vi "Open Workbook.vi"(7 "Create if does not exist? (T)":bool=TRUE, 8 "error in (no error)":errorcluster, 10 "File Name":path) -> (0 "error out":errorcluster, 3 "Workbook Reference Out":refnum<k24>)   [LabVIEW 2013]
uses:
  C:/PhaeronGit/LVNPOI/Resources/NPOI 2.1.1 dotnet2/NPOI.dll
  Resources/NPOI 2.1.1 dotnet2/NPOI.dll
  <vilib>/Utility/error.llb/Error Cluster From Error Code.vi
  <vilib>/ErrorRing/Error Ring.xnode
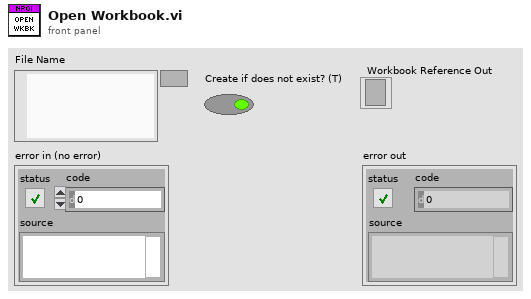
[diagram p1: front panel]
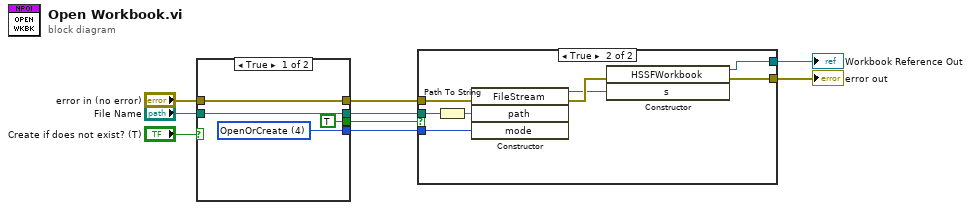
[diagram p0: block diagram]
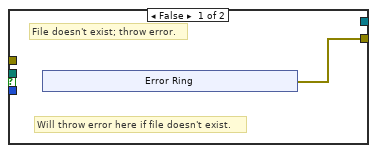
[diagram p2: hidden frame]
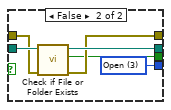
[diagram p3: hidden frame]
diagram:
  n1 = case shown="True" "Create if does not exist? (T)" {
    tunnel: [w13 w19] -> w7
    tunnel: [w12 w15] -> w6
    tunnel: "error in (no error)" -> [w12 w16]
    tunnel: [w11 w17] -> w4
    tunnel: "File Name" -> [w11 w18]
    tunnel: [TRUE ("file or folder exists?") w14] -> w1
    frame True {
      w13 = 4 items=["CreateNew"=1, "Create"=2, "Open"=3, "OpenOrCreate"=4, "Truncate"=5, "Append"=6] ("mode")
    }
    frame False {
      w19 = 3 items=["CreateNew"=1, "Create"=2, "Open"=3, "OpenOrCreate"=4, "Truncate"=5, "Append"=6] ("mode")
      n2 = call <vilib>:"Check if File or Folder Exists.vi"("error in (no error)"=w16, "path"=w18) -> ("error out"=w15:errorcluster, "file or folder exists?"=w14:bool, "dup path"=w17:path)  [unwired: 7 in]
    }
  }
  n3 = case shown="True" w1 {
    tunnel: [_ w30] -> w9
    tunnel: [w20 w29] -> w8
    tunnel: w7 -> [_ w28]
    tunnel: w6 -> [_ w27]
    tunnel: w4 -> [_ w26]
    frame False {
      # "File doesn't exist; throw error."
      # "Will throw error here if file doesn't exist."
      n4 = xnode "Error Ring"() -> ("error out"=w20:errorcluster)
    }
    frame True {
      n5 = Path To String(path=w26) -> (string=w32:string)
      n6 = constructor class="FileStream"(error in=w27, "path"=w32, "mode"=w28) -> (reference out=w25:refnum<k24>, error out=w31:errorcluster)  [unwired: 2 in, 3 out]
      n7 = constructor class="HSSFWorkbook"(error in=w31, "s"=w25) -> (reference out=w30:refnum<k24>, error out=w29:errorcluster)  [unwired: 2 in, 2 out]
    }
  }
  "Workbook Reference Out" <- w9
  "error out" <- w8
